vi "Analyze Data.vi"(8 "error in":errorcluster, 11 "PAS in":refnum<class "PAS.lvclass">) -> (0 "error out":errorcluster, 3 "PAS out":refnum<class "PAS.lvclass">)   [LabVIEW 2018, in "PAS Library.lvlib" / "PAS.lvclass"]
doc: "This is the core routine for PAS microphone data analysis. Here, the microphone data is retrieved from each of the cells. In both cases, the time domain signal will be transformed to the frequency domain. If the speaker is on (<B>Spk Pos</B> == TRUE), then the frequency domain signal will be squared to obtain the power and a Lorentzian will be fit to the data to retrieve the resonant characteristics of the cell. If the speaker is off (<B>Spk Pos</B> == FALSE), then the amplitude will be used to calculate the integrated area of the signal. In every case, the implementation has the ability to decimate the data for transmission of the waveforms over a network line."
uses:
  PAS.lvclass
  C:/Users/Labview/Documents/exscalabar_server/reusable/Instrument/Instrument.lvclass
  Data/Main/PAS Data.lvclass
  C:/Users/Labview/Documents/exscalabar_server/reusable/Data/Data.lvclass
  PAS.lvclass/PAS.ctl
  Instrument/Instrument.lvclass/Instrument.ctl
  Cell/PAS Cell.lvclass/PAS Cell.ctl
  Instrument/Read ExtCom.vi
  Instrument/Read Data.vi
  Cell/Read Mod Freq.vi
  Instrument/Write Data.vi
  Read Chirp.vi
  Get Speaker State.vi
  Data/Main/Read CellData.vi
  Data/Cell/Read f0.vi
  Read Cells.vi
  Data/Main/Write drive.vi
  Data/Main/Read filter.vi
  Cell/Read extParams.vi
  Write Cells.vi
  Data/Data.lvclass
  Data/Cell/PAS Cell Data.lvclass
  Cell/PAS Cell.lvclass
  Instrument/Instrument.lvclass
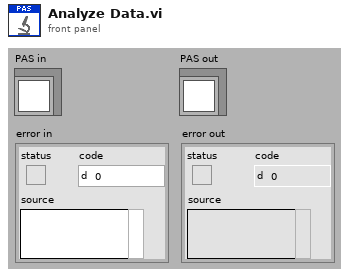
[diagram p1: front panel]
types:
  T1 = cluster{"tag":string, "section":string, "data":variant}
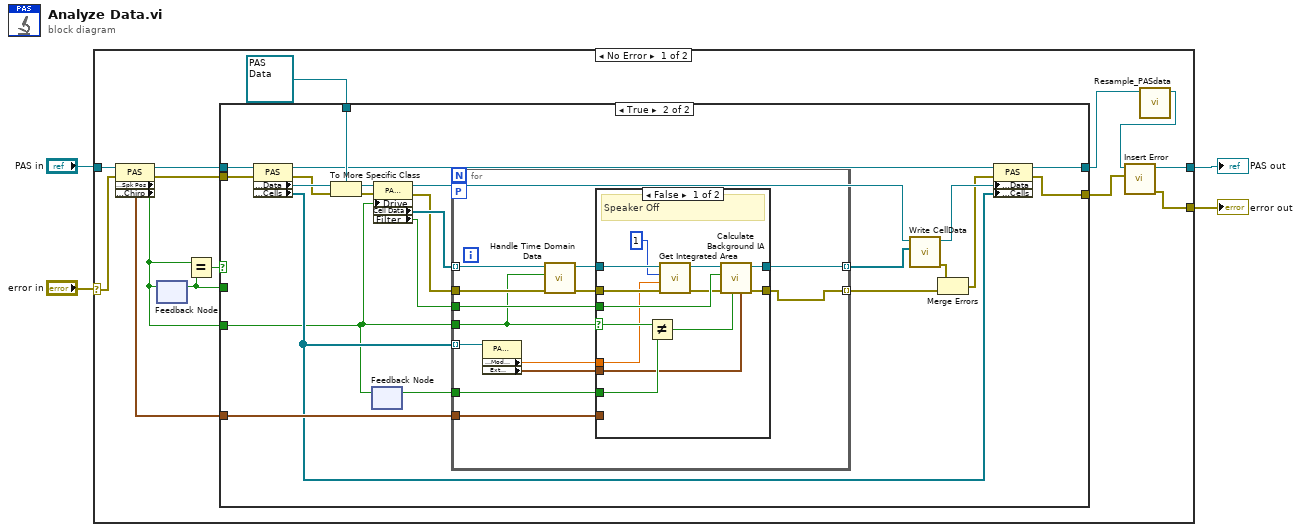
[diagram p0: block diagram]
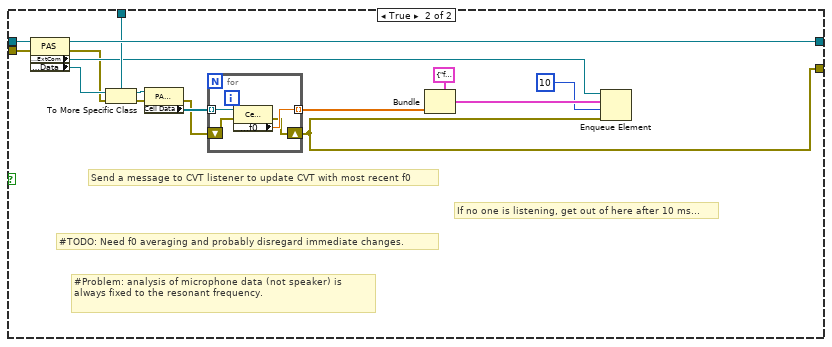
[diagram p3: hidden frame]
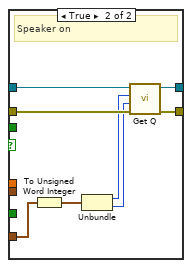
[diagram p4: hidden frame]
diagram:
  n1 = case shown="No Error" "error in" {
    selector: "error in" -> [w13 w105]
    tunnel: [w17 w105] -> w1
    tunnel: [w18 w104] -> w2
    tunnel: "PAS in" -> [w16 w104]
    frame No Error {
      n2 = property class="PAS"(reference=w16, error in=w13) -> (reference out=w15:refnum<class "PAS.lvclass">, error out=w14:errorcluster, "Data Access:Spk Pos"=w9:bool, "Data Access:Chirp"=w12:cluster{"f_center":dbl, "bandwidth":dbl})
      n3 = feedback-in #1(w9) -> ()
      n4 = feedback #1() -> (w7:bool)  [unwired: 1 in]
      n5 = Equal?(x=w9, y=w7) -> (x = y?=w10:bool)
      n6 = case shown="True" w10 {
        tunnel: [w21 w53] -> w6
        tunnel: w15 -> [w24 w67]
        tunnel: w14 -> [w23 w52]
        tunnel: w9 -> [_ w48]
        tunnel: w12 -> [_ w69]
        tunnel: [w22 w49] -> w11
        tunnel: refnum<class "PAS Data.lvclass"> refnum ("reference") -> [w20 w68]
        tunnel: w7 -> [w19 _]
        frame False {
          n7 = case shown="False" w19 {
            tunnel: w24 -> [w26 w42]
            tunnel: w23 -> [w25 w41]
            tunnel: [w25 w28] -> w22
            tunnel: [w26 w40] -> w21
            tunnel: w20 -> [_ w39]
            frame False {
            }
            frame True {
              # "If no one is listening, get out of here after 10 ms..."
              # "#Problem: analysis of microphone data (not speaker) is always fixed to the resonant frequency."
              # "#TODO: Need f0 averaging and probably disregard immediate changes."
              # "Send a message to CVT listener to update CVT with most recent f0"
              n8 = property class="PAS"(reference=w42, error in=w41) -> (reference out=w40:refnum<class "PAS.lvclass">, error out=w27:errorcluster, "Accessors:ExtCom"=w37:refnum<queue>, "Accessors:Data"=w38:refnum<class "Data.lvclass">)
              n9 = To More Specific Class(target class=w39, reference=w38, error in=w27) -> (specific class reference=w32:refnum<class "PAS Data.lvclass">, error out=w30:errorcluster)
              n10 = property class="PAS Data"(reference=w32, error in=w30) -> (error out=w29:errorcluster, "Cell Data"=w31:refnum<class "PAS Cell Data.lvclass">[])  [unwired: 1 out]
              n11 = for {
                tunnel: [w45] -> w35 mode=indexing
                tunnel: w31 -> [w46] mode=indexing
                shift-right: [w43] -> w28
                shift-left: w29 -> [w44]
                n12 = property class="Cell Data"(reference=w46, error in=w44) -> (error out=w43:errorcluster, "Accessors:f0"=w45:sgl)  [unwired: 1 out]
              }
              n13 = Bundle(cluster=T1 {"tag"="f0", "section"="pas.las", "data"=variant} ("element"), "data"=w35) -> (w34:T1)  [unwired: 2 in]
              n14 = Enqueue Element(queue=w37, element=w34, timeout in ms (-1)=10, error in (no error)=w28) -> ()  [unwired: 3 out]
            }
          }
        }
        frame True {
          n15 = property class="PAS"(reference=w67, error in=w52) -> (reference out=w55:refnum<class "PAS.lvclass">, error out=w51:errorcluster, "Accessors:Data"=w57:refnum<class "Data.lvclass">, "Data Access:Cells"=w54:refnum<class "PAS Cell.lvclass">[])
          n16 = To More Specific Class(target class=w68, reference=w57, error in=w51) -> (specific class reference=w59:refnum<class "PAS Data.lvclass">, error out=w58:errorcluster)
          n17 = feedback #2() -> (w47:bool)  [unwired: 1 in]
          n18 = feedback-in #2(w48) -> ()
          n19 = property class="PAS Data"(reference=w59, error in=w58, "Drive"=w48) -> (reference out=w62:refnum<class "PAS Data.lvclass">, error out=w61:errorcluster, "Cell Data"=w63:refnum<class "PAS Cell Data.lvclass">[], "Filter"=w60:bool)
          n20 = for {
            tunnel: w63 -> [w79] mode=indexing
            tunnel: [w70] -> w66 mode=indexing
            tunnel: [w71] -> w65 mode=indexing
            workers-P: _ -> [_]
            tunnel: w48 -> [w75]
            tunnel: w61 -> [w76]
            tunnel: w54 -> [w82] mode=indexing
            tunnel: w69 -> [w81]
            tunnel: w60 -> [w80]
            tunnel: w47 -> [w74]
            n21 = property class="PAS Cell"(reference=w82) -> ("Accessors:Mod Freq"=w72:sgl, "Ext Params"=w73:cluster{"slope":sgl, "zero":sgl})  [unwired: 1 in, 2 out]
            n22 = call "Handle Time Domain Data.vi"("error in"=w76, "Spkeaker On?"=w75, "Cell Data in"=w79) -> ("error out"=w77:errorcluster, "Cell Data out"=w78:refnum<class "PAS Cell Data.lvclass">)  [unwired: 7 in]
            n23 = case shown="False" w75 {
              selector: w75 -> [w92 _]
              tunnel: w78 -> [w91 w101]
              tunnel: w77 -> [w87 w100]
              tunnel: [w94 w103] -> w71
              tunnel: [w95 w102] -> w70
              tunnel: w73 -> [w84 _]
              tunnel: w81 -> [_ w97]
              tunnel: w80 -> [w93 _]
              tunnel: w74 -> [w86 _]
              tunnel: w72 -> [w85 _]
              frame False {
                # "Speaker Off"
                n24 = Not Equal?(x=w92, y=w86) -> (x != y?=w83:bool)
                n25 = call "Get Integrated Area.vi"("error in"=w87, "fmod"=w85, "p"=1 ("Integrated Area"), "PAS Cell Data in"=w91) -> ("error out"=w89:errorcluster, "PAS Cell Data out"=w90:refnum<class "PAS Cell Data.lvclass">)  [unwired: 6 in]
                n26 = call "Calculate Background IA.vi"("Fit Params"=w84, "Sw From Spk"=w83, "error in"=w89, "Filter"=w93, "Cell Data in"=w90) -> ("error out"=w94:errorcluster, "Cell Data out"=w95:refnum<class "PAS Cell Data.lvclass">)  [unwired: 5 in]
              }
              frame True {
                # "Speaker on"
                n27 = To Unsigned Word Integer(number=w97) -> (unsigned 16bit integer=w96:cluster{"f_center":u16, "bandwidth":u16})
                n28 = Unbundle(w96) -> ("f_center"=w99:u16, "bandwidth"=w98:u16)
                n29 = call "Get Q.vi"("error in"=w100, "Bandwidth"=w98, "f_center"=w99, "PAS Cell Data in"=w101) -> ("error out"=w103:errorcluster, "PAS Cell Data out"=w102:refnum<class "PAS Cell Data.lvclass">)  [unwired: 6 in]
              }
            }
          }
          n30 = call "Write CellData.vi"("CellData"=w66, "PAS Data in"=w62) -> ("error out"=w64:errorcluster, "PAS Data out"=w56:refnum<class "PAS Data.lvclass">)  [unwired: 8 in]
          n31 = Merge Errors(w64, w65) -> (w50:errorcluster)
          n32 = property class="PAS"(reference=w55, error in=w50, "Accessors:Data"=w56, "Data Access:Cells"=w54) -> (reference out=w53:refnum<class "PAS.lvclass">, error out=w49:errorcluster)
        }
      }
      n33 = call "Resample_PASdata.vi"("PAS in"=w6) -> ("PAS out"=w5:refnum<class "PAS.lvclass">)  [unwired: 9 in, 1 out]
      n34 = call "Insert Error.vi"("err"=w11, "Instrument in"=w5) -> ("error out"=w17:errorcluster, "Instrument out"=w18:refnum<class "PAS.lvclass">)  [unwired: 7 in, 1 out]
    }
    frame Error {
    }
  }
  "error out" <- w1
  "PAS out" <- w2
